vi "LVClass_Camera get image sequence.vi"(0 "Camera in":refnum<class "Camera.lvclass">, 5 "Image array":refnum<class "Image.lvclass">[](array[class]), 7 "remove background?":bool, 11 "error in (no error)":errorcluster) -> (4 "Camera out":refnum<class "Camera.lvclass">, 6 "Image array (dup)":refnum<class "Image.lvclass">[](array[class]), 15 "error out":errorcluster)   [LabVIEW 2020, in "Camera.lvclass"]
doc: "Ask camera for array_size captures and retrieve images array (Synchronous mode\n- Blocking).\n\n<B>CameraIn</B> : Camera object.\n<B>CameraOut</B> : Camera object.\n<B>image_array_size</B> : Captured sequence length (number of images).\n<B>image_array</B> : Captured sequence as image array."
uses:
  Camera.lvclass
  Image.lvclass
  Camera.lvclass/Camera.ctl
  LVClass_Image read Image Compat ptr.vi
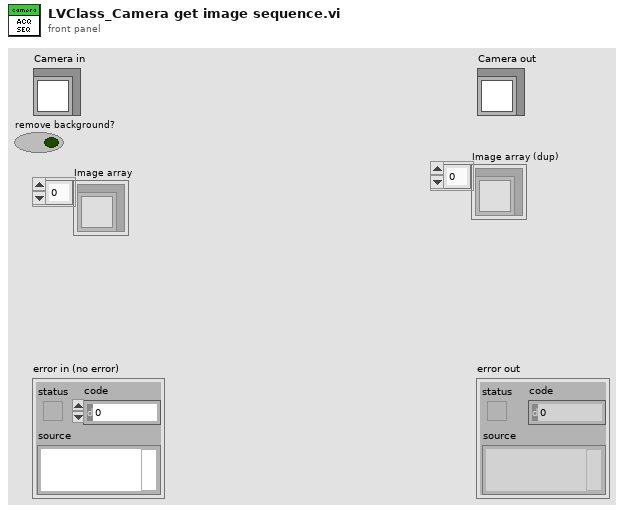
[diagram p1: front panel]
types:
  T1 = typedef "ClassID.ctl" = i64
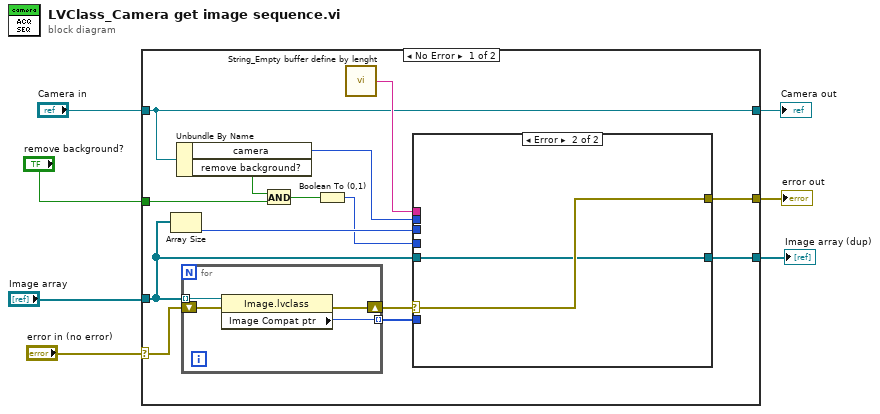
[diagram p0: block diagram]
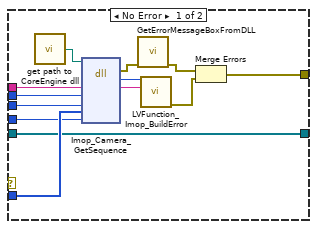
[diagram p2: hidden frame]
diagram:
  n1 = case shown="No Error" "error in (no error)" {
    selector: "error in (no error)" -> [w18 w43]
    tunnel: [w20 w43] -> w6
    tunnel: [w14 w42] -> w4
    tunnel: "Camera in" -> [w14 w42]
    tunnel: "Image array" -> [w12 w41]
    tunnel: [w15 w41] -> w2
    tunnel: "remove background?" -> [w10 _]
    frame No Error {
      n2 = Array Size(array=w12) -> (size(s)=w16:i32)
      n3 = Unbundle By Name(w14) -> ("camera"=w13:T1, "remove background?"=w9:bool)
      n4 = for {
        tunnel: w12 -> [w39] mode=indexing
        tunnel: [w40] -> w19 mode=indexing
        shift-right: [w37] -> w17
        shift-left: w18 -> [w38]
        n5 = property class="Image.lvclass"(reference=w39, error in=w38) -> (error out=w37:errorcluster, "Image Compat ptr"=w40:T1)  [unwired: 1 out]
      }
      n6 = And(x=w9, y=w10) -> (x .and. y?=w8:bool)
      n7 = Boolean To (0,1)(Boolean=w8) -> (0, 1=w11:i16)
      n8 = call "String_Empty buffer define by lenght.vi"() -> ("Empty buffer"=w21:string)  [unwired: 1 in]
      n9 = case shown="Error" w17 {
        selector: w17 -> [_ w36]
        tunnel: w21 -> [w34 _]
        tunnel: [w23 w36] -> w20
        tunnel: w13 -> [w31 _]
        tunnel: w19 -> [w30 _]
        tunnel: w16 -> [w27 _]
        tunnel: w12 -> [w26 w35]
        tunnel: [w26 w35] -> w15
        tunnel: w11 -> [w22 _]
        frame No Error {
          n10 = call "get path to CoreEngine dll.vi"() -> ("path to wavekit library"=w29:path)  [unwired: 14 in, 1 out]
          n11 = dll-call lib="D:/soft/HASO_v3/SVN_trunk/ImOpCoreEngine4_LV2011/DLLs/c_interface_vc100.dll" fn="Imop_Camera_GetSequence"(path in=w29, "message"=w34, "camera"=w31, "array_size"=w27, "HASO_image_array"=w30, "remove_background"=w22) -> (error out=w28:errorcluster, "return type"=w32:i32, "message"=w33:string)  [unwired: 6 in, 1 out]
          n12 = call "GetErrorMessageBoxFromDLL.vi"("error IN"=w28) -> ("error OUT"=w25:errorcluster)  [unwired: 10 in]
          n13 = call "LVFunction_Imop_BuildError.vi"("code"=w32, "String to Prepend to source (\"\")"=w33) -> ("error out"=w24:errorcluster)  [unwired: 13 in]
          n14 = Merge Errors(w25, w24) -> (w23:errorcluster)
        }
        frame Error {
        }
      }
    }
    frame Error {
    }
  }
  "error out" <- w6
  "Camera out" <- w4
  "Image array (dup)" <- w2
